vi "Get Menubar Color.vi"(11 "Results":T1) -> (3 "Fill Color":u32(colorbox)=13840175)   [LabVIEW 2020, in "Execution UI V2.lvclass"]
uses:
  Execution UI V2.lvclass
  Result Model/Statistics.ctl
  Result Model/Result Model.lvclass
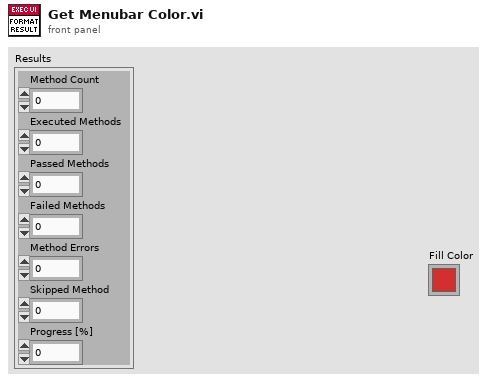
[diagram p1: front panel]
types:
  T1 = typedef "Result Model.lvclass/Statistics.ctl" = cluster{"Method Count":u32, "Executed Methods":u32, "Passed Methods":u32, "Failed Methods":u32, "Method Errors":u32, "Skipped Method":u32, "Progress [%]":dbl}
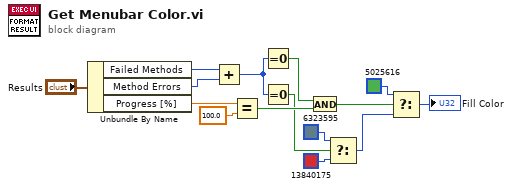
[diagram p0: block diagram]
diagram:
  n1 = Unbundle By Name("Results") -> ("Failed Methods"=w12:u32, "Method Errors"=w11:u32, "Progress [%]"=w14:dbl)
  n2 = Add(x=w12, y=w11) -> (x+y=w6:u32)
  n3 = Equal?(x=w14, y=100.0) -> (x = y?=w10:bool)
  n4 = Equal To 0?(x=w6) -> (x = 0?=w9:bool)
  n5 = Equal To 0?(x=w6) -> (x = 0?=w5:bool)
  n6 = And(x=w9, y=w10) -> (x .and. y?=w8:bool)
  n7 = Select(t=u32 6323595 ("Fill Color"), s=w5, f=u32 13840175 ("Fill Color")) -> (s? t:f=w2:u32)
  n8 = Select(t=u32 5025616 ("Fill Color"), s=w8, f=w2) -> (s? t:f=→"Fill Color":u32)
